vi "Cache.WriteError.vi"(8 "error in (no error)":errorcluster, 11 "Data in":T1) -> (0 "error out":errorcluster, 3 "Data out":T1)   [LabVIEW 2016]
uses:
  Global/ApplicationGlobal.vi
  Cache.Data.Status.ctl
  Cache.Data.Sets.ctl
  Cache.Data.ctl
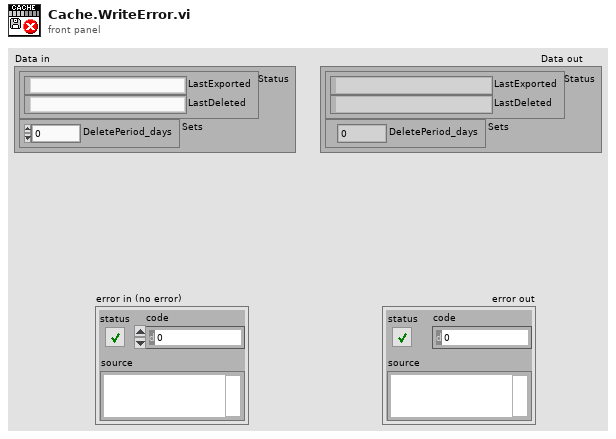
[diagram p1: front panel]
types:
  T1 = typedef "Cache.Data.ctl" = cluster{"Status":T2, "Sets":T3}
  T2 = typedef "Cache.Data.Status.ctl" = cluster{"LastExported":string, "LastDeleted":string}
  T3 = typedef "Cache.Data.Sets.ctl" = cluster{"DeletePeriod_days":dbl}
  T4 = enum16{"open", "open or create", "create or replace", "create", "open (read-only)"}
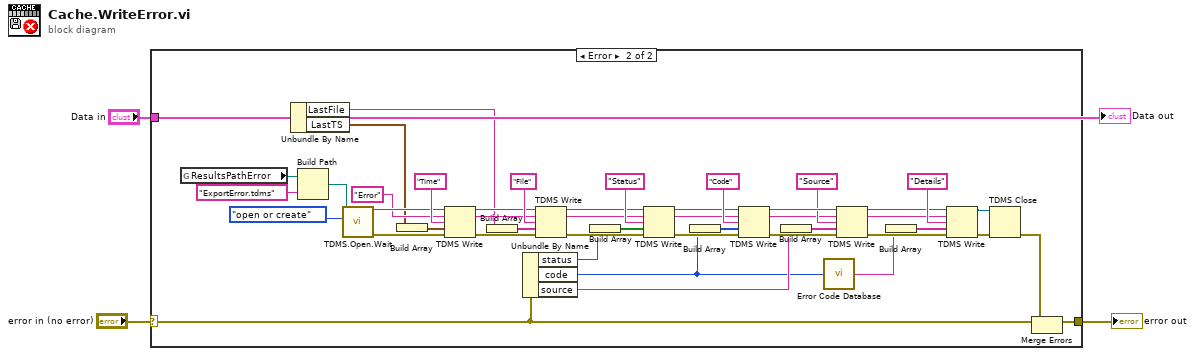
[diagram p0: block diagram]
diagram:
  n1 = case shown="Error" "error in (no error)" {
    selector: "error in (no error)" -> [w4 w12]
    tunnel: "Data in" -> [_ w7]
    tunnel: [w4 w13] -> w3
    frame No Error {
    }
    frame Error {
      n2 = global read "ApplicationGlobal.vi" "ResultsPathError"() -> (w10:path)
      n3 = Unbundle By Name(w7) -> ("LastFile"=w6:string, "LastTS"=w5:timestamp)
      n4 = Build Path(base path=w10, name or relative path="ExportError.tdms") -> (appended path=w37:path)
      n5 = call "TDMS.Open.Wait.vi"("operation (open read-only)"=T4."open or create", "file path"=w37) -> ("error out"=w31:errorcluster, "tdms file out"=w34:refnum<k34>)  [unwired: 8 in]
      n6 = Build Array(w5) -> (w30:timestamp[])
      n7 = TDMS Write(0:w34, 5:"Error" ("group name in (Untitled)"), 7:"Time" ("channel name"), 9:w30, 11:w31) -> (4:w33:refnum<k34>, 6:w24:string, 15:w32:errorcluster)  [unwired: 1 in, 1 out]
      n8 = Build Array(w6) -> (w29:string[])
      n9 = Unbundle By Name(w12) -> ("status"=w9:bool, "code"=w8:i32, "source"=w17:string)
      n10 = TDMS Write(0:w33, 5:w24, 7:"File" ("channel name"), 9:w29, 11:w32) -> (4:w39:refnum<k34>, 6:w27:string, 15:w36:errorcluster)  [unwired: 1 in, 1 out]
      n11 = Build Array(w9) -> (w49:bool[])
      n12 = TDMS Write(0:w39, 5:w27, 7:"Status" ("channel name"), 9:w49, 11:w36) -> (4:w46:refnum<k34>, 6:w26:string, 15:w45:errorcluster)  [unwired: 1 in, 1 out]
      n13 = Build Array(w8) -> (w44:i32[])
      n14 = TDMS Write(0:w46, 5:w26, 7:"Code" ("channel name"), 9:w44, 11:w45) -> (4:w43:refnum<k34>, 6:w25:string, 15:w42:errorcluster)  [unwired: 1 in, 1 out]
      n15 = Build Array(w17) -> (w28:string[])
      n16 = call <vilib>:"Error Code Database.vi"("Error Code"=w8) -> ("Error Text"=w15:string)
      n17 = TDMS Write(0:w43, 5:w25, 7:"Source" ("channel name"), 9:w28, 11:w42) -> (4:w20:refnum<k34>, 6:w18:string, 15:w19:errorcluster)  [unwired: 1 in, 1 out]
      n18 = Build Array(w15) -> (w16:string[])
      n19 = TDMS Write(0:w20, 5:w18, 7:"Details" ("channel name"), 9:w16, 11:w19) -> (4:w21:refnum<k34>, 15:w22:errorcluster)  [unwired: 1 in, 2 out]
      n20 = TDMS Close(8:w22, 11:w21) -> (0:w14:errorcluster)  [unwired: 1 out]
      n21 = Merge Errors(w12, w14) -> (w13:errorcluster)
    }
  }
  "error out" <- w3
  "Data out" <- "Data in"
